vi "initClass.vi"(8 "error in (no error)":errorcluster, 10 "input cluster":T1, 11 "GiaoTiepUART in":refnum<class "GiaoTiepUART.lvclass">) -> (0 "error out":errorcluster, 3 "GiaoTiepUART out":refnum<class "GiaoTiepUART.lvclass">)   [LabVIEW 2017, in "GiaoTiepUART.lvclass"]
uses:
  GiaoTiepUART.lvclass
  GiaoTiepUART.lvclass/GiaoTiepUART.ctl
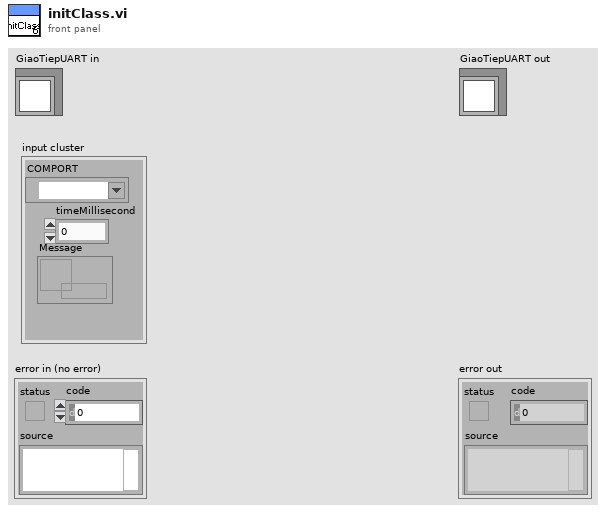
[diagram p1: front panel]
types:
  T1 = cluster{"COMPORT":refnum<visa-resource-name>, "timeMillisecond":dbl, "Message":refnum<queue>}
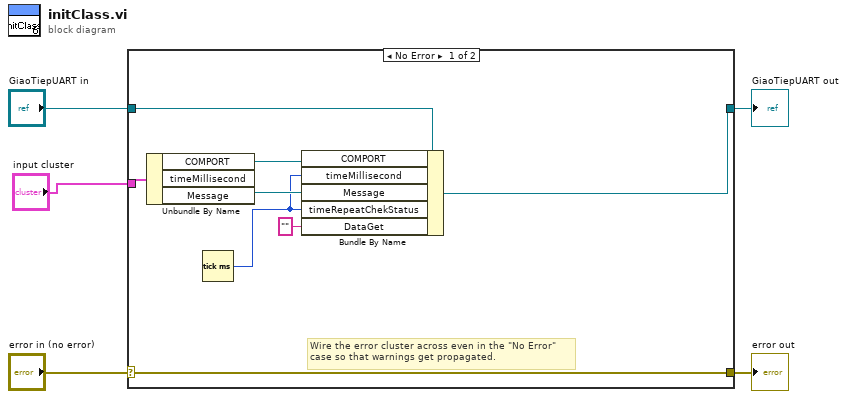
[diagram p0: block diagram]
diagram:
  n1 = case shown="No Error" "error in (no error)" {
    selector: "error in (no error)" -> [w13 w15]
    tunnel: [w13 w15] -> w4
    tunnel: [w11 w14] -> w2
    tunnel: "GiaoTiepUART in" -> [w12 w14]
    tunnel: "input cluster" -> [w10 _]
    frame No Error {
      # "Wire the error cluster across even in the \"No Error\"\ncase so that warnings get propagated."
      n2 = Unbundle By Name(w10) -> ("COMPORT"=w9:refnum<visa-resource-name>, "Message"=w8:refnum<queue>)  [unwired: 1 out]
      n3 = Tick Count (ms)() -> (millisecond timer value=w7:u32)
      n4 = Bundle By Name(cluster=w12, "COMPORT"=w9, "timeMillisecond"=w7, "Message"=w8, "timeRepeatChekStatus"=w7, "DataGet"="") -> (w11:refnum<class "GiaoTiepUART.lvclass">)
    }
    frame Error {
    }
  }
  "error out" <- w4
  "GiaoTiepUART out" <- w2
